vi "waveform_io.vi"() -> ()   [LabVIEW 2021]
uses:
  <vilib>/Waveform/WDTFileIO.llb/ Write Waveform to File.vi
  <vilib>/Waveform/WDTFileIO.llb/Read Waveform from File.vi
  <vilib>/Waveform/WDTFileIO.llb/Export Waveform To Spreadsheet File.vi
panel:
  out "Waveform Read From File":waveform(dbl)(graph)
  out "Waveform Written to File":waveform(dbl)(graph)
  in  "# of Points":i64
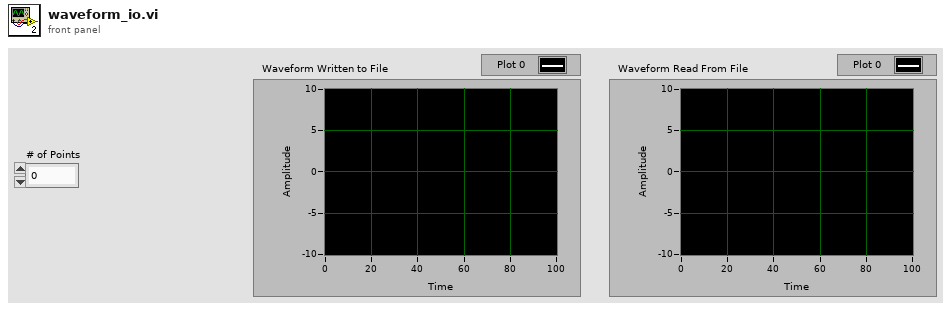
[diagram p1: front panel]
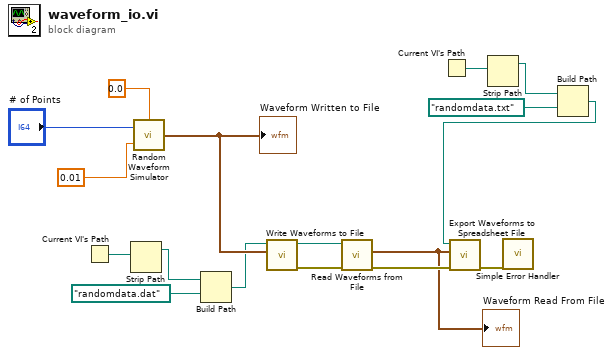
[diagram p0: block diagram]
diagram:
  n1 = Current VI's Path() -> (path=w13:path)
  n2 = Strip Path(path=w13) -> (stripped path=w14:path)  [unwired: 1 out]
  n3 = call "Random Waveform Simulator.vi"("Channel #"=0.0, "dt"=0.01, "# Points"="# of Points") -> ("waveform out"=w11:waveform(dbl))
  "Waveform Written to File" <- w11
  n4 = Build Path(base path=w14, name or relative path=path "randomdata.dat") -> (appended path=w10:path)
  n5 = call-poly <vilib>:"Write Waveforms to File.vi"("waveform"=w11, "file path (dialog if empty)"=w10) -> ("error out"=w9:errorcluster, "new file path (Not A Path if cancelled)"=w8:path)  [unwired: 8 in]
  n6 = call-poly <vilib>:"Read Waveforms from File.vi"("error in (no error)"=w9, "file path (dialog if empty)"=w8) -> ("error out"=w3:errorcluster, "first waveform in record"=w2:waveform(dbl))  [unwired: 4 in, 2 out]
  "Waveform Read From File" <- w2
  n7 = Current VI's Path() -> (path=w6:path)
  n8 = Strip Path(path=w6) -> (stripped path=w7:path)  [unwired: 1 out]
  n9 = Build Path(base path=w7, name or relative path=path "randomdata.txt") -> (appended path=w1:path)
  n10 = call-poly <vilib>:"Export Waveforms to Spreadsheet File.vi"("error in (no error)"=w3, "waveform"=w2, "file path (dialog if empty)"=w1) -> ("error out"=w4:errorcluster)  [unwired: 7 in, 1 out]
  n11 = call <vilib>:"Simple Error Handler.vi"("error in (no error)"=w4) -> ()  [unwired: 4 in, 5 out]
